vi "Loop Time.vi"() -> (0 "Time":u32)   [LabVIEW 2015]
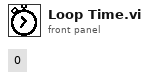
[diagram p1: front panel]
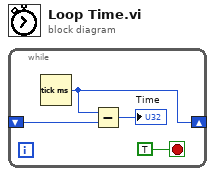
[diagram p0: block diagram]
diagram:
  n1 = while {
    shift-right: [w2] -> _
    shift-left: _ -> [w3]
    stop <- TRUE stop-if-true
    n2 = Tick Count (ms)() -> (millisecond timer value=w2:u32)
    n3 = Subtract(x=w2, y=w3) -> (x-y=→"Time":u32)
  }
